vi "Create Conditions.vi"(5 "Sequencing":refnum<class "MessageQ.lvclass">, 6 "Variables":refnum<class "Variables.lvclass">, 7 "VolatusAPI":refnum<class "VolatusAPI.lvclass">, 8 "error in (no error)":refnum<class "MultiErrors.lvclass">, 10 "Transition Config":refnum<class "Transition Config.lvclass">, 11 "Transition in":refnum<class "Transition.lvclass">) -> (0 "error out":refnum<class "MultiErrors.lvclass">, 3 "Transition out":refnum<class "Transition.lvclass">)   [LabVIEW 2020, in "VolatusSeq.lvlib" / "Transition.lvclass"]
uses:
  Transition.lvclass
  Transition.lvclass/Transition.ctl
  VolatusSeqConfig/Transition Config/Transition Config.lvclass
  Condition/Condition.lvclass
  Volatus/VolatusAPI/VolatusAPI.lvclass
  VolatusErrorUtilities/MultiErrors/MultiErrors.lvclass
  Volatus/MessageQ/MessageQ.lvclass
  Variables/Variables.lvclass
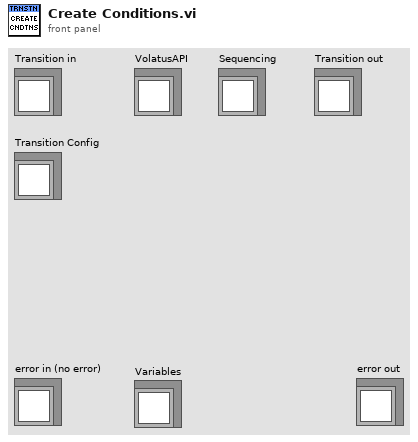
[diagram p1: front panel]
types:
  T1 = typedef "VolatusSeqConfig.lvlib/Condition Logic.ctl" = enum16{"All", "Any"}
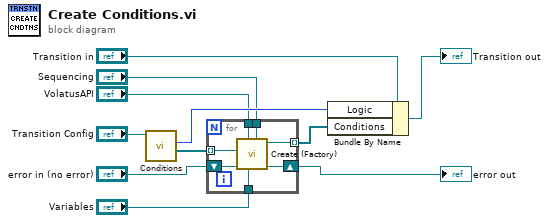
[diagram p0: block diagram]
diagram:
  n1 = call "Conditions.vi"("Transition Config in"="Transition Config") -> ("Conditions"=w7:refnum<class "Condition Config.lvclass">[], "Logic"=w8:T1)  [unwired: 9 in]
  n2 = for {
    tunnel: w7 -> [w18] mode=indexing
    tunnel: "VolatusAPI" -> [w17]
    tunnel: [w16] -> w5 mode=indexing
    shift-right: [w14] -> w3
    shift-left: "error in (no error)" -> [w15]
    tunnel: "Sequencing" -> [w13]
    tunnel: "Variables" -> [w12]
    n3 = call "Create (Factory).vi"("Sequencing"=w13, "Variables"=w12, "VolatusAPI"=w17, "error in (no error)"=w15, "Condition Config"=w18) -> ("error out"=w14:refnum<class "MultiErrors.lvclass">, "Condition out"=w16:refnum<class "Condition.lvclass">)  [unwired: 5 in]
  }
  "error out" <- w3
  n4 = Bundle By Name(cluster="Transition in", "Logic"=w8, "Conditions"=w5) -> (→"Transition out":refnum<class "Transition.lvclass">)
